vi "Drive Control Loop.vi"() -> ()   [LabVIEW 2019]
uses:
  .Team Code/Robot Global Data.vi
  <vilib>/Rock Robotics/WPI/ThirdParty/Phoenix-LabVIEW/Motor Controller/Controls/CTRE_Phoenix_MotorControl_ControlMode.ctl
  Calculations or utilities/Is command done typedef.ctl
  <vilib>/Rock Robotics/WPI/ThirdParty/Phoenix-LabVIEW/Pigeon IMU/CTRE_PigeonIMU_GetYPR.vi
panel:
  out "Gyro":dbl(graph)
  out "Drive Velocity":T1(graph)
  out "Drive Position":T2(graph)
  in  "Acceptable Position Error":dbl
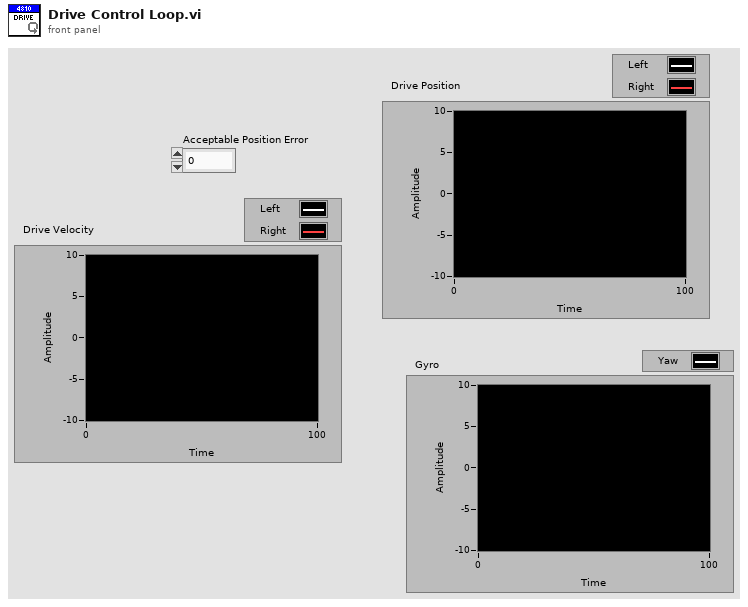
[diagram p1: front panel]
types:
  T1 = cluster{"Left Velocity (u/100ms)":i32, "Right Velocity (u/100ms)":i32}
  T2 = cluster{"Left Position (u)":i32, "Right Position (u)":i32}
  T3 = typedef "CTRE_PigeonIMU_DeviceRef.ctl" = cluster{"DeviceStatus":errorcluster, "Device Number":u8, "Type":T4, "Device ID":u32, "Handle":u64, "UsageFrame":u32, "Library Path":path}
  T4 = typedef "CTRE_PigeonIMU_ConnectionType.ctl" = u32
  T5 = typedef "WPI_MotorControlDeviceRef.ctl" = cluster{"DeviceStatus":errorcluster, "Type":T6, "PWM":cluster{"PWM Channel":T7, "DeadBand":T8}, "CAN":cluster{"Device Number":u8, "SetOutput VI Ref":variant, "GetOutput VI Ref":variant, "Enable VI Ref":variant, "Disable VI Ref":variant, "Data":variant}, "Invert":bool, "DIO PWM":cluster{"PWM \"Enable\" Channel":T7, "DIOChannel":T9, "PWM Rate":dbl}}
  T6 = typedef "WPI_MotorControlType.ctl" = enum16{"PWM", "CAN", "DIO PWM"}
  T7 = typedef "FPGA_DIOPWMChannel.ctl" = enum8{"PWM 0", "PWM 1", "PWM 2", "PWM 3", "PWM 4", "PWM 5", "PWM 6", "PWM 7", "PWM 8", "PWM 9", "PWM MXP 0", "PWM MXP 1", "PWM MXP 2", "PWM MXP 3", "PWM MXP 4", "PWM MXP 5", "PWM MXP 6", "PWM MXP 7", "PWM MXP 8", "PWM MXP 9", "Invalid"}
  T8 = typedef "WPI_PWMDeadband.ctl" = cluster{"Name":string, "maxPositivePwm":i32, "minPositivePwm":i32, "centerPwm":i32, "maxNegativePwm":i32, "minNegativePwm":i32, "angularRange":u16}
  T9 = typedef "FPGA_DIOChannel.ctl" = enum8{"DIO 0", "DIO 1", "DIO 2", "DIO 3", "DIO 4", "DIO 5", "DIO 6", "DIO 7", "DIO 8", "DIO 9", "DIO MXP 0", "DIO MXP 1", "DIO MXP 2", "DIO MXP 3", "DIO MXP 4", "DIO MXP 5", "DIO MXP 6", "DIO MXP 7", "DIO MXP 8", "DIO MXP 9", "DIO MXP 10", "DIO MXP 11", "DIO MXP 12", "DIO MXP 13", "DIO MXP 14", "DIO MXP 15", "SPI Port CS1", "SPI Port CS2", "SPI Port CS3", "SPI Port MISO", "SPI Port MOSI", "Invalid"}
  T10 = typedef "Is command done typedef.ctl" = cluster{"Done?":bool, "Timestamp [ms]":dbl}
  T11 = typedef "Drive Command Typedef.ctl" = cluster{"Drive Mode":T12, "LeftValue[%]/ relative Distance[u]":dbl, "Right Motor Value[%]":dbl, "Timestamp [ms]":dbl}
  T12 = typedef "Drive Mode Typedef.ctl" = enum16{"Disabled", "Auto-align", "Drive Distance", "Turn to angle", "Driver"}
  T13 = typedef "CTRE_Phoenix_MotorControl_ControlMode.ctl" = u16
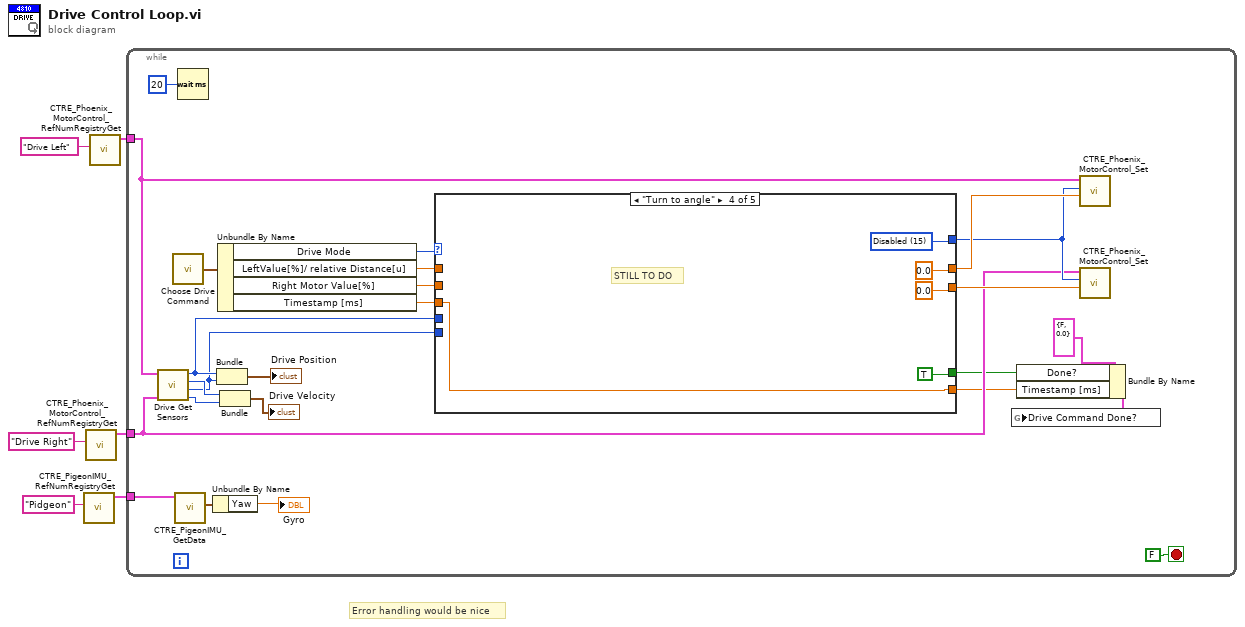
[diagram p0: block diagram]
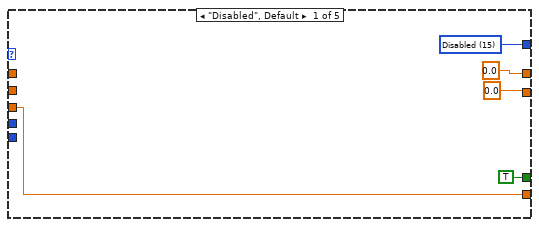
[diagram p2: hidden frame]
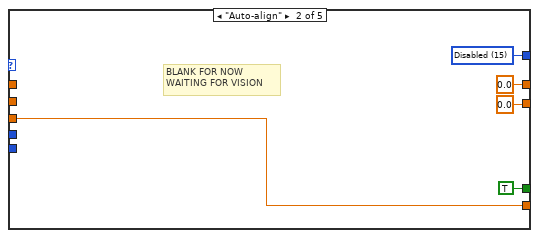
[diagram p3: hidden frame]
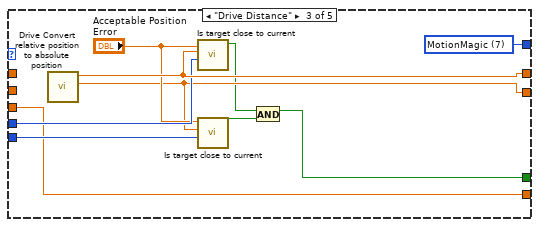
[diagram p4: hidden frame]
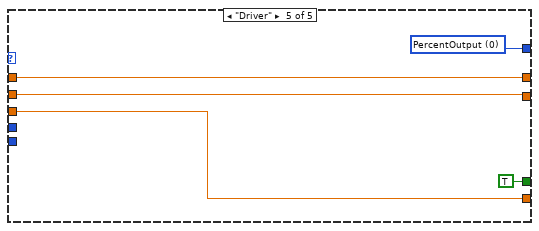
[diagram p5: hidden frame]
diagram:
  # "Error handling would be nice"
  n1 = call <vilib>:"CTRE_PigeonIMU_RefNumRegistryGet.vi"("refnum name"="Pidgeon") -> ("PigeonIMUDevRef"=w1:T3)  [unwired: 9 in, 1 out]
  n2 = call <vilib>:"CTRE_Phoenix_MotorControl_RefNumRegistryGet.vi"("refnum name"="Drive Right") -> ("PhoenixMotorControlDevRef"=w3:T5)  [unwired: 9 in, 1 out]
  n3 = call <vilib>:"CTRE_Phoenix_MotorControl_RefNumRegistryGet.vi"("refnum name"="Drive Left") -> ("PhoenixMotorControlDevRef"=w4:T5)  [unwired: 9 in, 1 out]
  n4 = while {
    tunnel: w4 -> [w22]
    tunnel: w3 -> [w21]
    tunnel: w1 -> [w9]
    stop <- FALSE stop-if-true
    n5 = call "Drive Get Sensors.vi"("Right Drive DevRef"=w21, "Left Drive DevRef"=w22) -> ("Right Velocity (u/100ms)"=w19:i32, "Right Position (u)"=w15:i32, "Left Velocity (u/100ms)"=w20:i32, "Left Position (u)"=w16:i32)  [unwired: 6 in]
    n6 = call "Choose Drive Command.vi"() -> ("Current Drive Command"=w25:T11)  [unwired: 1 in]
    n7 = call-poly <vilib>:"CTRE_PigeonIMU_GetData.vi"("PigeonIMUDevRef"=w9) -> ("Yaw Pitch Roll"=w8:cluster{"Yaw":dbl, "Pitch":dbl, "Roll":dbl})  [unwired: 8 in, 2 out]
    n8 = Wait (ms)(milliseconds to wait=u32 20) -> ()  [unwired: 1 out]
    n9 = Unbundle By Name(w8) -> ("Yaw"=→"Gyro":dbl)
    n10 = Bundle("Left Position (u)"=w16, "Right Position (u)"=w15) -> (→"Drive Position":T2)  [unwired: 1 in]
    n11 = Unbundle By Name(w25) -> ("Drive Mode"=w29:T12, "LeftValue[%]/ relative Distance[u]"=w13:dbl, "Right Motor Value[%]"=w12:dbl, "Timestamp [ms]"=w11:dbl)
    n12 = Bundle("Left Velocity (u/100ms)"=w20, "Right Velocity (u/100ms)"=w19) -> (→"Drive Velocity":T1)  [unwired: 1 in]
    n13 = case shown="\"Turn to angle\"" w29 {
      tunnel: [w36 w39 w51 w56 w61] -> w26
      tunnel: [0.0 ("Output") 0.0 ("LeftValue[%]/ relative Distance[u]") w50 0.0 ("LeftValue[%]/ relative Distance[u]") w59] -> w28
      tunnel: [0.0 ("Output") 0.0 ("LeftValue[%]/ relative Distance[u]") w47 0.0 ("LeftValue[%]/ relative Distance[u]") w58] -> w27
      tunnel: w16 -> [_ _ w49 _ _]
      tunnel: w15 -> [_ _ w46 _ _]
      tunnel: [TRUE TRUE w43 TRUE TRUE] -> w14
      tunnel: w13 -> [_ _ _ _ w59]
      tunnel: w12 -> [_ _ _ _ w58]
      tunnel: [w32 w40 w42 w52 w57] -> w10
      tunnel: w11 -> [w32 w40 w42 w52 w57]
      frame "Disabled", Default {
        w36 = T13 15 items=["PercentOutput"=0, "Position"=1, "Velocity"=2, "Current"=3, "Follower"=5, "MotionProfile"=6, "MotionMagic"=7, "MotionProfileArc"=10, "Disabled"=15] ("Control Mode")
      }
      frame "Auto-align" {
        w39 = T13 15 items=["PercentOutput"=0, "Position"=1, "Velocity"=2, "Current"=3, "Follower"=5, "MotionProfile"=6, "MotionMagic"=7, "MotionProfileArc"=10, "Disabled"=15] ("Control Mode")
        # "BLANK FOR NOW\nWAITING FOR VISION"
      }
      frame "Drive Distance" {
        w51 = T13 7 items=["PercentOutput"=0, "Position"=1, "Velocity"=2, "Current"=3, "Follower"=5, "MotionProfile"=6, "MotionMagic"=7, "MotionProfileArc"=10, "Disabled"=15] ("Control Mode")
        n14 = call "Drive Convert relative position to absolute position.vi"() -> ("Right Target Position"=w47:dbl, "Left Target Position"=w50:dbl)  [unwired: 10 in]
        n15 = call "Is target close to current.vi"("Current Position"=w49, "Target Position"=w50, "Acceptable Error"="Acceptable Position Error") -> ("Acceptable"=w44:bool)  [unwired: 8 in]
        n16 = call "Is target close to current.vi"("Current Position"=w46, "Target Position"=w47, "Acceptable Error"="Acceptable Position Error") -> ("Acceptable"=w45:bool)  [unwired: 8 in]
        n17 = And(x=w44, y=w45) -> (x .and. y?=w43:bool)
      }
      frame "Turn to angle" {
        w56 = T13 15 items=["PercentOutput"=0, "Position"=1, "Velocity"=2, "Current"=3, "Follower"=5, "MotionProfile"=6, "MotionMagic"=7, "MotionProfileArc"=10, "Disabled"=15] ("Control Mode")
        # "STILL TO DO"
      }
      frame "Driver" {
        w61 = T13 0 items=["PercentOutput"=0, "Position"=1, "Velocity"=2, "Current"=3, "Follower"=5, "MotionProfile"=6, "MotionMagic"=7, "MotionProfileArc"=10, "Disabled"=15] ("Control Mode")
      }
    }
    n18 = Bundle By Name(cluster=T10 {"Done?"=FALSE, "Timestamp [ms]"=0.0} ("Command Done?"), "Done?"=w14, "Timestamp [ms]"=w10) -> (w24:T10)
    n19 = global write "Robot Global Data.vi" "Drive Command Done?"(w24) -> ()
    n20 = call <vilib>:"CTRE_Phoenix_MotorControl_Set.vi"("Output"=w28, "Control Mode"=w26, "PhoenixMotorControlDevRef"=w22) -> ()  [unwired: 7 in, 2 out]
    n21 = call <vilib>:"CTRE_Phoenix_MotorControl_Set.vi"("Output"=w27, "Control Mode"=w26, "PhoenixMotorControlDevRef"=w21) -> ()  [unwired: 7 in, 2 out]
  }
